vi "Local Search_IRH3TPopulation.vi"(8 "error in (no error)":errorcluster, 10 "OSSP_Problem in":refnum<class "OSSP_Problem.lvclass">, 11 "GA in":refnum<class "GA.lvclass">) -> (0 "error out":errorcluster, 2 "OSSP_Problem out":refnum<class "OSSP_Problem.lvclass">, 3 "GA out":refnum<class "GA.lvclass">)   [LabVIEW 2013]
uses:
  Classes/GA.lvclass
  Classes/OSSP_Problem.lvclass
  Classes/OSSP_Problem.lvclass/OSSP_Problem.ctl
  Classes/GA.lvclass/GA.ctl
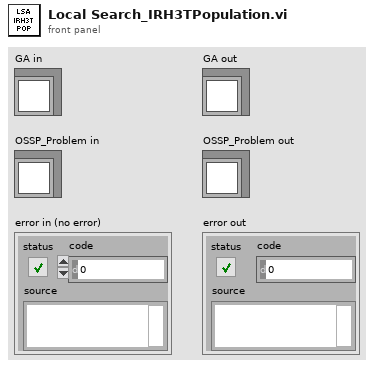
[diagram p1: front panel]
types:
  T1 = typedef "Solution_GA.ctl" = cluster{"Schedule":u16[], "Fitness":u16, "Fitness Valid?":bool}
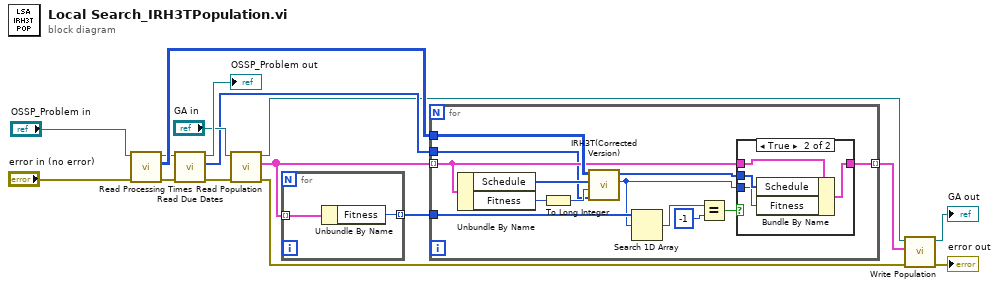
[diagram p0: block diagram]
diagram:
  n1 = call "Read Processing Times.vi"("error in (no error)"="error in (no error)", "OSSP_Problem in"="OSSP_Problem in") -> ("error out"=w8:errorcluster, "Processing Times"=w10:u16[][], "OSSP_Problem out"=w9:refnum<class "OSSP_Problem.lvclass">)  [unwired: 7 in]
  n2 = call "Read Due Dates.vi"("error in (no error)"=w8, "OSSP_Problem in"=w9) -> ("error out"=w6:errorcluster, "Due Dates"=w7:u16[], "OSSP_Problem out"=→"OSSP_Problem out":refnum<class "OSSP_Problem.lvclass">)  [unwired: 7 in]
  n3 = call "Read Population.vi"("error in (no error)"=w6, "GA in"="GA in") -> ("error out"=w4:errorcluster, "Population"=w2:T1[], "GA out"=w5:refnum<class "GA.lvclass">)  [unwired: 7 in]
  n4 = for {
    tunnel: w2 -> [w18] mode=indexing
    tunnel: [w17] -> w1 mode=indexing
    n5 = Unbundle By Name(w18) -> ("Fitness"=w17:u16)
  }
  n6 = for {
    tunnel: w10 -> [w31]
    tunnel: w7 -> [w24]
    tunnel: w2 -> [w30] mode=indexing
    tunnel: [w29] -> w3 mode=indexing
    tunnel: w1 -> [w23]
    n7 = Unbundle By Name(w30) -> ("Schedule"=w27:u16[], "Fitness"=w26:u16)
    n8 = To Long Integer(number=w26) -> (32bit integer=w25:i32)
    n9 = call "IRH3T(Corrected Version).vi"("Due Dates"=w24, "Initial Tardiness"=w25, "Schedule 2B Improved"=w27, "Proocessing Times  (Machines x Jobs)"=w31) -> ("Total Tardiness"=w19:u16, "IRH3T (Reordered) Schedule Out"=w28:u16[])  [unwired: 5 in, 1 out]
    n10 = Search 1D Array(1D array=w23, element=w19) -> (index of element=w22:i32)  [unwired: 1 in]
    n11 = Equal?(x=w22, y=-1) -> (x = y?=w20:bool)
    n12 = case shown="True" w20 {
      tunnel: w30 -> [w32 w36]
      tunnel: [w32 w35] -> w29
      tunnel: w28 -> [_ w34]
      tunnel: w19 -> [_ w33]
      frame False {
      }
      frame True {
        n13 = Bundle By Name(cluster=w36, "Schedule"=w34, "Fitness"=w33) -> (w35:T1)
      }
    }
  }
  n14 = call "Write Population.vi"("error in (no error)"=w4, "Population"=w3, "GA in"=w5) -> ("error out"=→"error out":errorcluster, "GA out"=→"GA out":refnum<class "GA.lvclass">)  [unwired: 7 in]
